vi "ROSToQueue.vi"(4 "ROS":T1={"topic port"=0, "Node"="", "topic"="", "type"="", "node port"=0, "error "={"status"=FALSE, "code"=0, "source"=""}, "Direction"=enum."Node", "Update (ms)"=1, "FIFO size"=1}, 5 "Name":enum16{"topic", "node"}(ring)) -> (0 "error out":errorcluster, 1 "queue":refnum<queue>)   [LabVIEW 2014]
doc: "Places ROS definitions onto the queue"
uses:
  <userlib>/ROS for LabVIEW Software.lnk/ROS/Code/SubVIs/_ROSControl.ctl
  <userlib>/ROS for LabVIEW Software.lnk/ROS/Code/SubVIs/_ROSDirection.ctl
  <userlib>/ROS for LabVIEW Software.lnk/ROS/Code/_ROSDefinition.vi
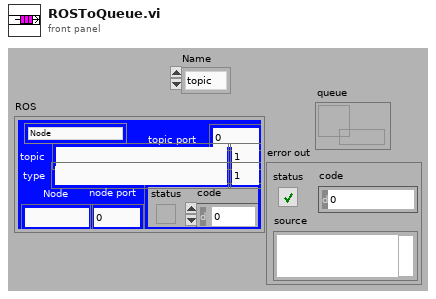
[diagram p1: front panel]
types:
  T1 = typedef "_ROSControl.ctl" = cluster{"topic port":u16, "Node":string, "topic":string, "type":string, "node port":u16, "error ":errorcluster, "Direction":T2, "Update (ms)":u16, "FIFO size":u16}
  T2 = typedef "_ROSDirection.ctl" = enum16{"Node", "Publisher", "Subscriber", "ServiceClient", "ServiceProvider"}
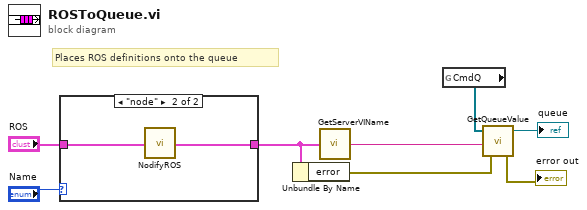
[diagram p0: block diagram]
diagram:
  # "Places ROS definitions onto the queue"
  n1 = case shown="\"node\"" "Name" {
    tunnel: [w9 w10] -> w3
    tunnel: "ROS" -> [w9 w11]
    frame "topic", Default {
    }
    frame "node" {
      n2 = call <userlib>:"NodifyROS.vi"("ROS in"=w11) -> ("ROS out"=w10:T1)
    }
  }
  n3 = Unbundle By Name(w3) -> ("error"=w2:errorcluster)
  n4 = call <userlib>:"GetServerVIName.vi"("ROS"=w3) -> ("vi name"=w7:string)
  n5 = global read "_ROSDefinition.vi" "CmdQ"() -> (w1:refnum<queue>[])
  n6 = call <userlib>:"GetQueueValue.vi"("error in"=w2, "vi name"=w7, "Q"=w1) -> ("error out"=→"error out":errorcluster, "Queue out"=→"queue":refnum<queue>)  [unwired: 1 in]
